vi "svx_Commit Hardware Settings (DAQmx).vi"(0 "acquisition task in":T1={"AI device settings"={"AI DAQmx TaskID"="", "response"=[]}, "acquisition type"=enum."Finite", "measurement settings"={"AI sampling frequency"=51200.0, "AO sampling frequency"=51200.0, "AI block size"=0, "AO block Size"=0, "block duration [ms]"=100.0, "number of AI channels"=0, "device propagation delay [samples]"=0.0, "DUT propagation time [s]"=0.0}, "settling settings"={"settle time"=0.015599999576807022, "settle cycles"=5}, "integration settings"={"integration time"=0.015599999576807022, "integration cycles"=5}, "AO device settings"={"AO DAQmx taskID"="", "excitation"=[]}, "acquisition accounting"={"initial read size [samples]"=0, "read offset [samples]"=0, "read length [samples]"=0, "blocks to settle [samples]"=0, "min delay until transition [samples]"=0}, "frequency range"={"start frequency"=0.015599999576807022, "stop frequency"=5.0}, "block type"=enum."Initialize", "source settings"={"signal type"=enum."Dual tone (IMD)", "frequency"=0.0, "total amplitude"=0.0, "frequencies"=[1.0], "relative amplitudes"=[1.0], "offset"=1.0, "total amplitude list"=[1.0], "ramping rate"=0.0}, "chirp settings"={"amplitude"=0.0, "frequency range"={"start (Hz)"=20.0, "stop (Hz)"=20000.0, "frequency spacing"=enum."Logarithmic"}, "sampling info"={"Fs"=50000.0, "chirp duration [s]"=3.0}, "initial states"={"frequency [Hz]"=20.0, "phase [rad]"=0.0, "elapsed time [s]"=0.0}, "frequency slope"=0.0, "maximum harmonic"=0, "prefix len [samples]"={"integer"=0, "fractional"=0.0}}} {"chirp settings"."frequency slope" format="%.2f"; "chirp settings"."prefix len [samples]"."fractional" format="%.2p"; "chirp settings"."initial states"."elapsed time [s]" format="%.2f"; "chirp settings"."initial states"."phase [rad]" format="%.2f"; "chirp settings"."initial states"."frequency [Hz]" format="%.2f"; "chirp settings"."sampling info"."chirp duration [s]" format="%.2f"; "chirp settings"."sampling info"."Fs" format="%.2p"; "chirp settings"."frequency range"."stop (Hz)" format="%.2f"; "chirp settings"."frequency range"."start (Hz)" format="%.2f"; "chirp settings"."amplitude" format="%.2f"; "source settings"."total amplitude" format="%.2f"; "source settings"."relative amplitudes" format="%.2f"; "source settings"."frequencies" format="%.2f"; "source settings"."total amplitude list" format="%.2f"; "source settings"."ramping rate" format="%.4f"; "source settings"."offset" format="%.2f"; "source settings"."frequency" format="%.2f"; "frequency range"."stop frequency" format="%.2f"; "frequency range"."start frequency" format="%.2f"; "AO device settings"."excitation"."AO channel settings"."terminal config" items=["Default"=-1, "Differential"=10106, "Pseudodifferential"=12529]; "AI device settings"."response"."AI channel settings"."DSA channel settings"."IEPE current [mA]" min=0.0 max=20.0 format="%.1f"; "AI device settings"."response"."AI channel settings"."DSA channel settings"."coupling" items=["AC"=10045, "DC"=10050, "GND"=10066]; "AI device settings"."response"."AI channel settings"."min value [V]" format="%.2f"; "AI device settings"."response"."AI channel settings"."terminal config" items=["Default"=-1, "RSE"=10083, "NRSE"=10078, "Differential"=10106, "Pseudodifferential"=12529]; "AI device settings"."response"."AI channel settings"."max value [V]" format="%.2f"; "integration settings"."integration time" format="%.2p"; "settling settings"."settle time" format="%.2p"; "measurement settings"."DUT propagation time [s]" format="%.2f"; "measurement settings"."AO sampling frequency" format="%.2f"; "measurement settings"."AI sampling frequency" format="%.2f"}, 11 "error in (no error)":errorcluster, 12 "block size limits":T5={"minimum block size"=50, "maximum block size"=131072}) -> (4 "acquisition task out":T1={"AI device settings"={"AI DAQmx TaskID"="", "response"=[{"AI physical channel"="Dev1/ai0", "AI channel settings"={"max value [V]"=10.0, "min value [V]"=10.0, "terminal config"=-1, "DSA channel settings"={"coupling"=10045, "enable IEPE excitation"=FALSE, "IEPE current [mA]"=4.0}}}]}, "acquisition type"=enum."Finite", "measurement settings"={"AI sampling frequency"=0.0, "AO sampling frequency"=0.0, "AI block size"=0, "AO block Size"=0, "block duration [ms]"=100.0, "number of AI channels"=0, "device propagation delay [samples]"=0.0, "DUT propagation time [s]"=0.0}, "settling settings"={"settle time"=0.015599999576807022, "settle cycles"=5}, "integration settings"={"integration time"=0.015599999576807022, "integration cycles"=5}, "AO device settings"={"AO DAQmx taskID"="", "excitation"=[{"AO physical channel"="Dev1/ao0", "AO channel settings"={"maximum value (10 V)"=10.0, "minimum value (10 V)"=-10.0, "terminal config"=-1}}]}, "acquisition accounting"={"initial read size [samples]"=0, "read offset [samples]"=0, "read length [samples]"=0, "blocks to settle [samples]"=0, "min delay until transition [samples]"=0}, "frequency range"={"start frequency"=-1.0, "stop frequency"=-1.0}, "block type"=enum."Initialize", "source settings"={"signal type"=enum."Sine wave", "frequency"=0.0, "total amplitude"=0.0, "frequencies"=[1.0], "relative amplitudes"=[1.0], "offset"=1.0, "total amplitude list"=[1.0], "ramping rate"=0.0}, "chirp settings"={"amplitude"=0.0, "frequency range"={"start (Hz)"=20.0, "stop (Hz)"=20000.0, "frequency spacing"=enum."Logarithmic"}, "sampling info"={"Fs"=50000.0, "chirp duration [s]"=3.0}, "initial states"={"frequency [Hz]"=20.0, "phase [rad]"=0.0, "elapsed time [s]"=0.0}, "frequency slope"=0.0, "maximum harmonic"=0, "prefix len [samples]"={"integer"=0, "fractional"=0.0}}} {"chirp settings"."frequency slope" format="%.2f"; "chirp settings"."prefix len [samples]"."fractional" format="%.2p"; "chirp settings"."initial states"."elapsed time [s]" format="%.2f"; "chirp settings"."initial states"."phase [rad]" format="%.2f"; "chirp settings"."initial states"."frequency [Hz]" format="%.2f"; "chirp settings"."sampling info"."chirp duration [s]" format="%.2f"; "chirp settings"."sampling info"."Fs" format="%.2p"; "chirp settings"."frequency range"."stop (Hz)" format="%.2f"; "chirp settings"."frequency range"."start (Hz)" format="%.2f"; "chirp settings"."amplitude" format="%.2f"; "source settings"."total amplitude" format="%.2f"; "source settings"."relative amplitudes" format="%.2f"; "source settings"."frequencies" format="%.2f"; "source settings"."total amplitude list" format="%.2f"; "source settings"."ramping rate" format="%.4f"; "source settings"."offset" format="%.2f"; "source settings"."frequency" format="%.2f"; "frequency range"."stop frequency" format="%.2f"; "frequency range"."start frequency" format="%.2f"; "AO device settings"."excitation"."AO channel settings"."terminal config" items=["Default"=-1, "Differential"=10106, "Pseudodifferential"=12529]; "AI device settings"."response"."AI channel settings"."DSA channel settings"."IEPE current [mA]" min=0.0 max=20.0 format="%.1f"; "AI device settings"."response"."AI channel settings"."DSA channel settings"."coupling" items=["AC"=10045, "DC"=10050, "GND"=10066]; "AI device settings"."response"."AI channel settings"."min value [V]" format="%.2f"; "AI device settings"."response"."AI channel settings"."terminal config" items=["Default"=-1, "RSE"=10083, "NRSE"=10078, "Differential"=10106, "Pseudodifferential"=12529]; "AI device settings"."response"."AI channel settings"."max value [V]" format="%.2f"; "integration settings"."integration time" format="%.2p"; "settling settings"."settle time" format="%.2p"; "measurement settings"."DUT propagation time [s]" format="%.2f"; "measurement settings"."AO sampling frequency" format="%.2f"; "measurement settings"."AI sampling frequency" format="%.2f"}, 13 "measurements per second":dbl format="%.2f", 14 "actual sample rate":dbl format="%.2f", 15 "error out":errorcluster)   [LabVIEW 2017]
doc: "This example VI commits the analog input and output tasks to perform an audio measurement on a DUT. Before calling <B>SVXMPL_Commit Hardware Settings (DAQmx).vi</B>, you should initialize and configure the measurment task using <B>SVXMPL_Initialize (DAQmx).vi</B>, <B>SVXMPL_Configure Source (DAQmx).vi</B>, <B>SVXMPL_Configure Measurement.vi</B>, and (if needed) <B>SVXMPL_Override DAQmx Parameters.vi</B>.\n\nThe only configuration input for this VI is the <B>block size limits</B> cluster. The block size, in samples, is dependent on input selections from <B>SVXMPL_Configure Measurement.vi</B> and <B>SVXMPL_Override DAQmx Parameters.vi</B>. If the block size defined in the task lies outside the <B>block size limits</B> it will be coerced into this range.\n\nThe VI returns the actual hardware sampling rate in samples per second as well as the time interval required for each integration period in the measurement."
uses:
  <vilib>/addons/Sound and Vibration/Example Support/Audio/DAQmx/svx_Acquisition Task (DAQmx).ctl
  <vilib>/addons/_NISVFA/_Shared subVIs/Controls/svc_Channel Settings.ctl
  <vilib>/addons/_NISVFA/_Shared subVIs/Controls/svc_DSA Channel Settings.ctl
  <vilib>/addons/_NISVFA/_Generation/subVIs/sv_Chirp Settings.ctl
  <vilib>/addons/_NISVFA/_Generation/SoundVib_Generation.lvlib
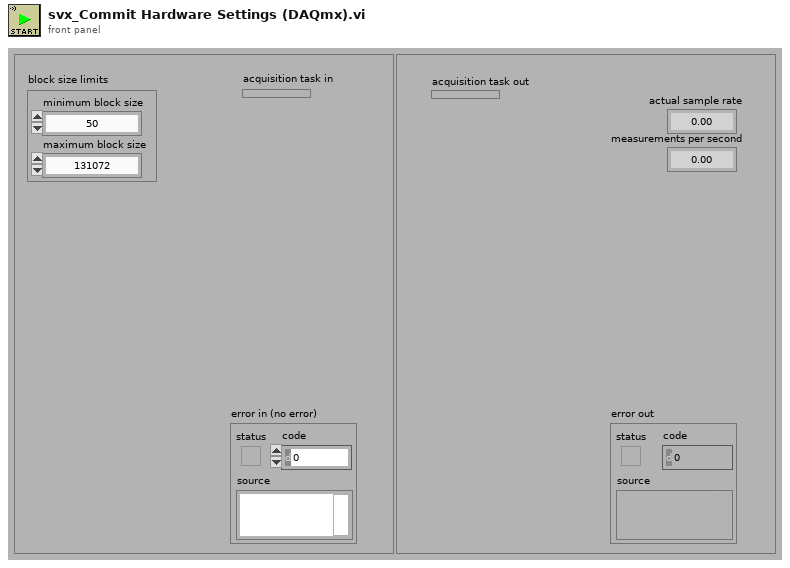
[diagram p1: front panel]
types:
  T1 = typedef "svx_Acquisition Task (DAQmx).ctl" = cluster{"AI device settings":cluster{"AI DAQmx TaskID":refnum<k21>, "response":cluster{"AI physical channel":tag, "AI channel settings":T2}[]}, "acquisition type":enum16{"Finite", "Averaged", "Settled", "Amplitude Sweep", "Stepped Frequency Sweep", "Continuous Frequency Sweep"}, "measurement settings":cluster{"AI sampling frequency":dbl, "AO sampling frequency":dbl, "AI block size":i32, "AO block Size":i32, "block duration [ms]":dbl, "number of AI channels":i32, "device propagation delay [samples]":dbl, "DUT propagation time [s]":dbl}, "settling settings":cluster{"settle time":dbl, "settle cycles":i32}, "integration settings":cluster{"integration time":dbl, "integration cycles":i32}, "AO device settings":cluster{"AO DAQmx taskID":refnum<k21>, "excitation":cluster{"AO physical channel":tag, "AO channel settings":cluster{"maximum value (10 V)":dbl, "minimum value (10 V)":dbl, "terminal config":i32}}[]}, "acquisition accounting":cluster{"initial read size [samples]":i32, "read offset [samples]":i32, "read length [samples]":i32, "blocks to settle [samples]":i32, "min delay until transition [samples]":i32}, "frequency range":cluster{"start frequency":dbl, "stop frequency":dbl}, "block type":enum16{"Initialize", "Settle", "Integrate"}, "source settings":cluster{"signal type":enum16{"Sine wave", "Dual tone (IMD)", "Multitone", "Chirp", "Frequency flat chirp", "Uniform white noise", "Gaussian white noise", "Pink noise", "PRN", "Continuous swept-sine"}, "frequency":dbl, "total amplitude":dbl, "frequencies":dbl[], "relative amplitudes":dbl[], "offset":dbl, "total amplitude list":dbl[], "ramping rate":dbl}, "chirp settings":T4}
  T2 = typedef "svc_Channel Settings.ctl" = cluster{"max value [V]":dbl, "min value [V]":dbl, "terminal config":i32, "DSA channel settings":T3}
  T3 = typedef "svc_DSA Channel Settings.ctl" = cluster{"coupling":i32, "enable IEPE excitation":bool, "IEPE current [mA]":dbl}
  T4 = typedef "SoundVib_Generation.lvlib/sv_Chirp Settings.ctl" = cluster{"amplitude":dbl, "frequency range":cluster{"start (Hz)":dbl, "stop (Hz)":dbl, "frequency spacing":enum16{"Linear", "Logarithmic"}}, "sampling info":cluster{"Fs":dbl, "chirp duration [s]":dbl}, "initial states":cluster{"frequency [Hz]":dbl, "phase [rad]":dbl, "elapsed time [s]":dbl}, "frequency slope":dbl, "maximum harmonic":i32, "prefix len [samples]":cluster{"integer":u32, "fractional":dbl}}
  T5 = cluster{"minimum block size":i32, "maximum block size":i32}
  T6 = enum16{"Finite", "Averaged", "Settled", "Amplitude Sweep", "Stepped Frequency Sweep", "Continuous Frequency Sweep"}
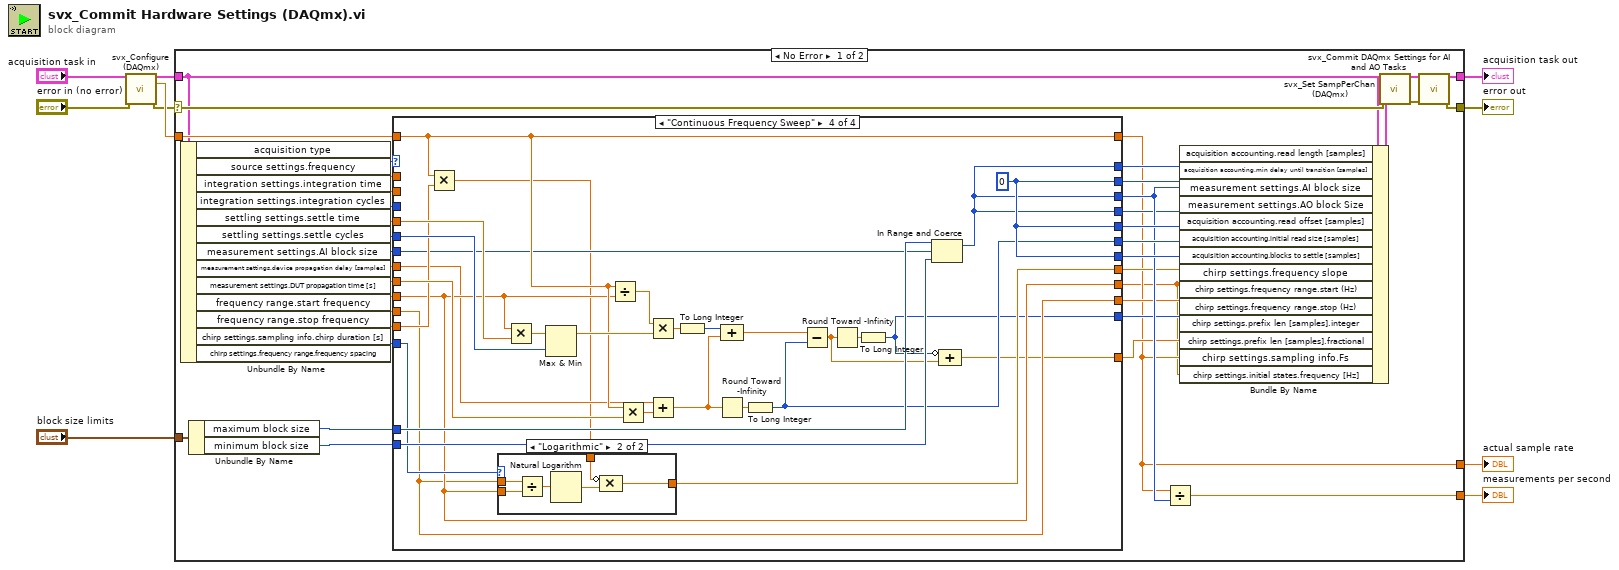
[diagram p0: block diagram]
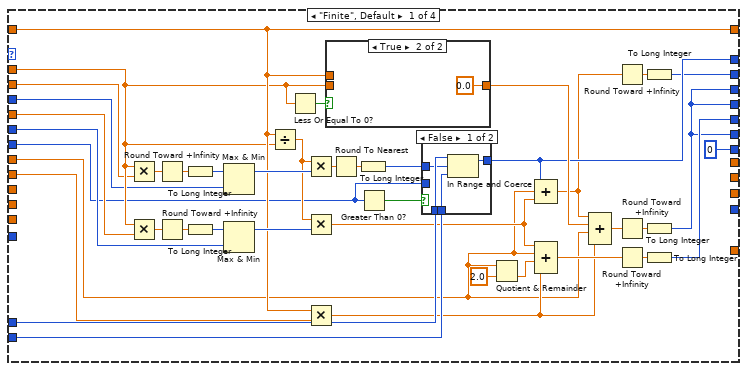
[diagram p2: hidden frame]
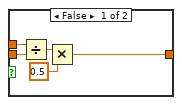
[diagram p4: hidden frame]
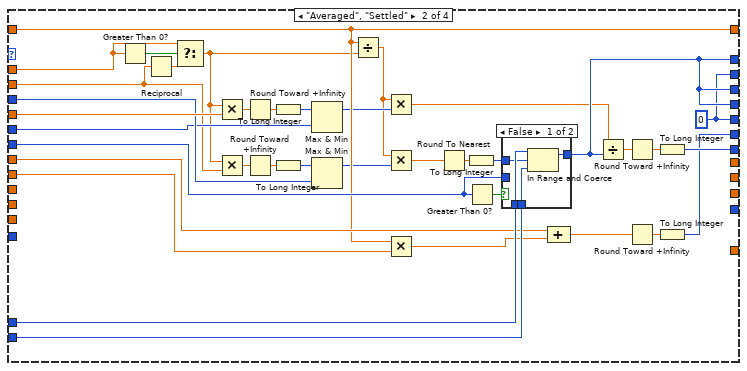
[diagram p5: hidden frame]
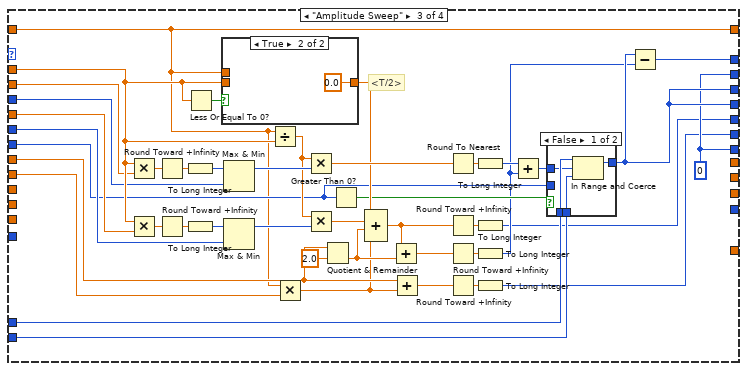
[diagram p7: hidden frame]
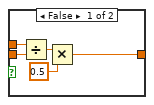
[diagram p9: hidden frame]
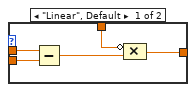
[diagram p10: hidden frame]
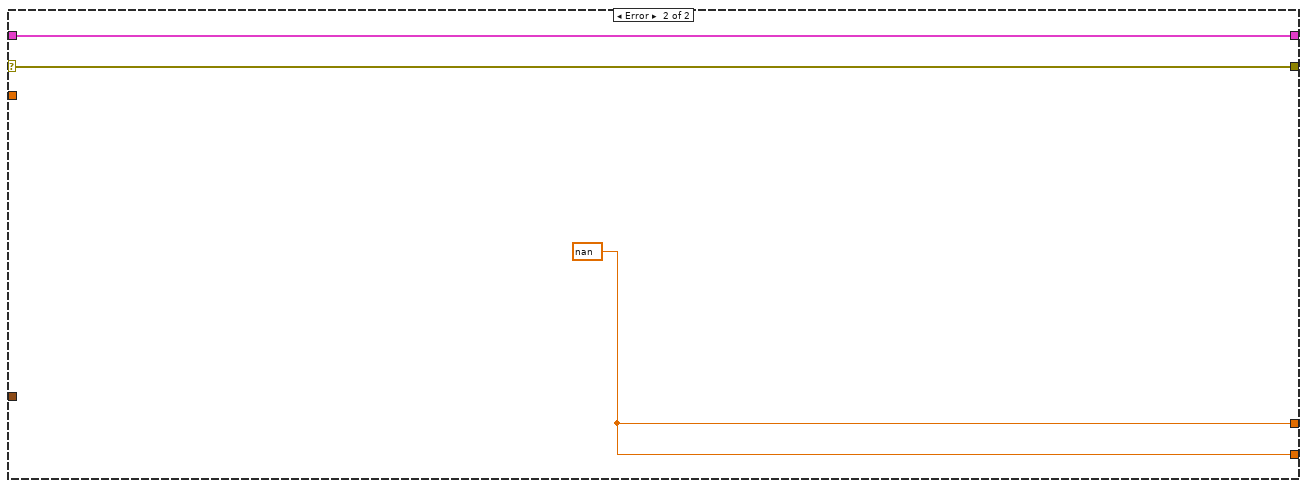
[diagram p11: hidden frame]
diagram:
  n1 = call <vilib>:"svx_Configure (DAQmx).vi"("acquisition task in"="acquisition task in", "error in (no error)"="error in (no error)") -> ("acquisition task out"=w4:T1, "actual scan rate"=w3:dbl, "error out"=w2:errorcluster)  [unwired: 11 in]
  n2 = case shown="No Error" w2 {
    selector: w2 -> [w27 w238]
    tunnel: w4 -> [w26 w240]
    tunnel: [w23 w240] -> w1
    tunnel: [w21 w238] -> w9
    tunnel: w3 -> [w30 _]
    tunnel: "block size limits" -> [w38 _]
    tunnel: [w31 w239] -> w6
    tunnel: [w12 w239] -> w5
    frame No Error {
      n3 = Unbundle By Name(w26) -> ("acquisition type"=w32:T6, "source settings.frequency"=w48:dbl, "integration settings.integration time"=w47:dbl, "integration settings.integration cycles"=w46:i32, "settling settings.settle time"=w45:dbl, "settling settings.settle cycles"=w44:i32, "measurement settings.AI block size"=w43:i32, "measurement settings.device propagation delay [samples]"=w42:dbl, "measurement settings.DUT propagation time [s]"=w41:dbl, "frequency range.start frequency"=w20:dbl, "frequency range.stop frequency"=w19:dbl, "chirp settings.sampling info.chirp duration [s]"=w18:dbl, "chirp settings.frequency range.frequency spacing"=w17:enum16{"Linear", "Logarithmic"})
      n4 = Unbundle By Name(w38) -> ("maximum block size"=w40:i32, "minimum block size"=w39:i32)
      n5 = case shown="\"Continuous Frequency Sweep\"" w32 {
        tunnel: w30 -> [w72 w113 w156 w217]
        tunnel: w48 -> [w68 w107 w167 _]
        tunnel: w47 -> [w67 w101 w166 _]
        tunnel: w46 -> [w66 w115 w165 _]
        tunnel: w45 -> [w65 w116 w164 w224]
        tunnel: w44 -> [w64 w114 w163 w223]
        tunnel: w43 -> [w63 w127 w162 w199]
        tunnel: w42 -> [w49 w132 w161 w209]
        tunnel: w41 -> [w62 w131 w160 w222]
        tunnel: w40 -> [w70 w134 w159 w221]
        tunnel: w39 -> [w69 w133 w158 w220]
        tunnel: [w72 w113 w156 w217] -> w12
        tunnel: [w71 w125 w157 w211] -> w37
        tunnel: [w56 w123 w154 w212] -> w36
        tunnel: [w53 w125 w155 w211] -> w29
        tunnel: [w53 w125 w155 w211] -> w28
        tunnel: [w58 w123 w145 w212] -> w35
        tunnel: [w53 w103 w151 w207] -> w34
        tunnel: [0 ("acquisition accounting.min delay until transition [samples]") w128 w154 w212] -> w33
        tunnel: w20 -> [_ _ _ w213]
        tunnel: w19 -> [_ _ _ w210]
        tunnel: w18 -> [_ _ _ w216]
        tunnel: w17 -> [_ _ _ w215]
        tunnel: [_ _ _ w214] -> w16
        tunnel: [_ _ _ w213] -> w11
        tunnel: [_ _ _ w210] -> w15
        tunnel: [_ _ _ w204] -> w13
        tunnel: [_ _ _ w198] -> w14
        frame "Finite", Default {
          n6 = Multiply(x=w68, y=w67) -> (x*y=w80:dbl)
          n7 = Multiply(x=w68, y=w65) -> (x*y=w78:dbl)
          n8 = Round Toward +Infinity(x=w80) -> (ceil(x): smallest int >= x=w81:dbl)
          n9 = Round Toward +Infinity(x=w78) -> (ceil(x): smallest int >= x=w77:dbl)
          n10 = To Long Integer(number=w81) -> (32bit integer=w82:i32)
          n11 = To Long Integer(number=w77) -> (32bit integer=w76:i32)
          n12 = Max & Min(x=w82, y=w66) -> (max(x,y)=w79:i32)  [unwired: 1 out]
          n13 = Max & Min(x=w76, y=w64) -> (max(x,y)=w75:i32)  [unwired: 1 out]
          n14 = Divide(x=w72, y=w68) -> (x/y=w74:dbl)
          n15 = Less Or Equal To 0?(x=w68) -> (x <= 0?=w89:bool)
          n16 = Multiply(x=w74, y=w79) -> (x*y=w85:dbl)
          n17 = Multiply(x=w74, y=w75) -> (x*y=w52:dbl)
          n18 = Multiply(x=w72, y=w62) -> (x*y=w51:dbl)
          n19 = case shown="True" w89 {
            tunnel: [w95 0.0] -> w84
            tunnel: w72 -> [w98 _]
            tunnel: w68 -> [w96 _]
            frame False {
              n20 = Divide(x=w98, y=w96) -> (x/y=w99:dbl)
              n21 = Multiply(x=w99, y=0.5) -> (x*y=w95:dbl)
            }
            frame True {
            }
          }
          n22 = Round To Nearest(number=w85) -> (nearest integer value=w86:dbl)
          n23 = To Long Integer(number=w86) -> (32bit integer=w88:i32)
          n24 = Greater Than 0?(x=w63) -> (x > 0?=w87:bool)
          n25 = case shown="False" w87 {
            tunnel: w88 -> [w91 _]
            tunnel: w63 -> [_ w94]
            tunnel: [w90 w94] -> w71
            tunnel: w70 -> [w93 _]
            tunnel: w69 -> [w92 _]
            frame False {
              n26 = In Range and Coerce(upper limit=w93, x=w91, lower limit=w92) -> (coerced(x)=w90:i32)  [unwired: 1 out]
            }
            frame True {
            }
          }
          n27 = Quotient & Remainder(x=w49, y=2.0) -> (floor(x/y)=w73:dbl)  [unwired: 1 out]
          n28 = Compound Arithmetic op=ADD(w71, w49, w52) -> (w50:dbl)
          n29 = Compound Arithmetic op=ADD(w52, w49, w73, w51) -> (w59:dbl)
          n30 = Compound Arithmetic op=ADD(w50, w84, w49, w51) -> (w54:dbl)
          n31 = Round Toward +Infinity(x=w50) -> (ceil(x): smallest int >= x=w57:dbl)
          n32 = Round Toward +Infinity(x=w54) -> (ceil(x): smallest int >= x=w55:dbl)
          n33 = Round Toward +Infinity(x=w59) -> (ceil(x): smallest int >= x=w60:dbl)
          n34 = To Long Integer(number=w57) -> (32bit integer=w56:i32)
          n35 = To Long Integer(number=w55) -> (32bit integer=w53:i32)
          n36 = To Long Integer(number=w60) -> (32bit integer=w58:i32)
        }
        frame "Averaged", "Settled" {
          w123 = 0
          n37 = Greater Than 0?(x=w107) -> (x > 0?=w109:bool)
          n38 = Reciprocal(x=w101) -> (1/x=w106:dbl)
          n39 = Select(t=w107, s=w109, f=w106) -> (s? t:f=w108:dbl)
          n40 = Multiply(x=w108, y=w116) -> (x*y=w119:dbl)
          n41 = Multiply(x=w108, y=w101) -> (x*y=w120:dbl)
          n42 = Round Toward +Infinity(x=w119) -> (ceil(x): smallest int >= x=w118:dbl)
          n43 = Round Toward +Infinity(x=w120) -> (ceil(x): smallest int >= x=w121:dbl)
          n44 = To Long Integer(number=w118) -> (32bit integer=w117:i32)
          n45 = To Long Integer(number=w121) -> (32bit integer=w122:i32)
          n46 = Max & Min(x=w117, y=w114) -> (max(x,y)=w112:i32)  [unwired: 1 out]
          n47 = Max & Min(x=w122, y=w115) -> (max(x,y)=w111:i32)  [unwired: 1 out]
          n48 = Divide(x=w113, y=w108) -> (x/y=w110:dbl)
          n49 = Multiply(x=w110, y=w112) -> (x*y=w124:dbl)
          n50 = Multiply(x=w110, y=w111) -> (x*y=w126:dbl)
          n51 = Multiply(x=w113, y=w131) -> (x*y=w102:dbl)
          n52 = Round To Nearest(number=w126) -> (nearest integer value=w135:dbl)
          n53 = To Long Integer(number=w135) -> (32bit integer=w137:i32)
          n54 = Greater Than 0?(x=w127) -> (x > 0?=w136:bool)
          n55 = case shown="False" w136 {
            tunnel: w137 -> [w139 _]
            tunnel: w127 -> [_ w142]
            tunnel: [w138 w142] -> w125
            tunnel: w134 -> [w141 _]
            tunnel: w133 -> [w140 _]
            frame False {
              n56 = In Range and Coerce(upper limit=w141, x=w139, lower limit=w140) -> (coerced(x)=w138:i32)  [unwired: 1 out]
            }
            frame True {
            }
          }
          n57 = Compound Arithmetic op=ADD(w132, w102) -> (w104:dbl)
          n58 = Divide(x=w124, y=w125) -> (x/y=w129:dbl)
          n59 = Round Toward +Infinity(x=w129) -> (ceil(x): smallest int >= x=w130:dbl)
          n60 = Round Toward +Infinity(x=w104) -> (ceil(x): smallest int >= x=w105:dbl)
          n61 = To Long Integer(number=w130) -> (32bit integer=w128:i32)
          n62 = To Long Integer(number=w105) -> (32bit integer=w103:i32)
        }
        frame "Amplitude Sweep" {
          w154 = 0 ("acquisition accounting.min delay until transition [samples]")
          # "<T/2>"
          n63 = Multiply(x=w167, y=w166) -> (x*y=w179:dbl)
          n64 = Multiply(x=w167, y=w164) -> (x*y=w177:dbl)
          n65 = Round Toward +Infinity(x=w179) -> (ceil(x): smallest int >= x=w180:dbl)
          n66 = Round Toward +Infinity(x=w177) -> (ceil(x): smallest int >= x=w176:dbl)
          n67 = To Long Integer(number=w180) -> (32bit integer=w181:i32)
          n68 = To Long Integer(number=w176) -> (32bit integer=w175:i32)
          n69 = Less Or Equal To 0?(x=w167) -> (x <= 0?=w185:bool)
          n70 = case shown="True" w185 {
            tunnel: [w191 0.0] -> w171
            tunnel: w156 -> [w194 _]
            tunnel: w167 -> [w192 _]
            frame False {
              n71 = Divide(x=w194, y=w192) -> (x/y=w195:dbl)
              n72 = Multiply(x=w195, y=0.5) -> (x*y=w191:dbl)
            }
            frame True {
            }
          }
          n73 = Max & Min(x=w181, y=w165) -> (max(x,y)=w178:i32)  [unwired: 1 out]
          n74 = Max & Min(x=w175, y=w163) -> (max(x,y)=w174:i32)  [unwired: 1 out]
          n75 = Divide(x=w156, y=w167) -> (x/y=w173:dbl)
          n76 = Multiply(x=w156, y=w160) -> (x*y=w143:dbl)
          n77 = Multiply(x=w173, y=w178) -> (x*y=w183:dbl)
          n78 = Multiply(x=w173, y=w174) -> (x*y=w144:dbl)
          n79 = Quotient & Remainder(x=w161, y=2.0) -> (floor(x/y)=w168:dbl)  [unwired: 1 out]
          n80 = Greater Than 0?(x=w162) -> (x > 0?=w169:bool)
          n81 = Compound Arithmetic op=ADD(w171, w144, w168, w143) -> (w146:dbl)
          n82 = Add(x=w146, y=w168) -> (x+y=w149:dbl)
          n83 = Add(x=w161, y=w143) -> (x+y=w152:dbl)
          n84 = Round To Nearest(number=w183) -> (nearest integer value=w184:dbl)
          n85 = Round Toward +Infinity(x=w146) -> (ceil(x): smallest int >= x=w147:dbl)
          n86 = Round Toward +Infinity(x=w149) -> (ceil(x): smallest int >= x=w150:dbl)
          n87 = Round Toward +Infinity(x=w152) -> (ceil(x): smallest int >= x=w153:dbl)
          n88 = To Long Integer(number=w184) -> (32bit integer=w172:i32)
          n89 = To Long Integer(number=w147) -> (32bit integer=w145:i32)
          n90 = To Long Integer(number=w150) -> (32bit integer=w148:i32)
          n91 = To Long Integer(number=w153) -> (32bit integer=w151:i32)
          n92 = Add(x=w172, y=w148) -> (x+y=w170:i32)
          n93 = case shown="False" w169 {
            tunnel: w170 -> [w187 _]
            tunnel: w162 -> [_ w190]
            tunnel: [w186 w190] -> w155
            tunnel: w159 -> [w189 _]
            tunnel: w158 -> [w188 _]
            frame False {
              n94 = In Range and Coerce(upper limit=w189, x=w187, lower limit=w188) -> (coerced(x)=w186:i32)  [unwired: 1 out]
            }
            frame True {
            }
          }
          n95 = Subtract(x=w155, y=w148) -> (x-y=w157:i32)
        }
        frame "Continuous Frequency Sweep" {
          w212 = 0 ("acquisition accounting.min delay until transition [samples]")
          n96 = Multiply(x=w217, y=w216) -> (x*y=w197:dbl)
          n97 = case shown="\"Logarithmic\"" w215 {
            tunnel: w210 -> [w230 w237]
            tunnel: w197 -> [w228 w234]
            tunnel: w213 -> [w231 w233]
            tunnel: [w227 w232] -> w214
            frame "Linear", Default {
              n98 = Subtract(x=w230, y=w231) -> (x-y=w229:dbl)
              n99 = Compound Arithmetic op=MULTIPLY(invert w228, w229) -> (w227:dbl)
            }
            frame "Logarithmic" {
              n100 = Divide(x=w237, y=w233) -> (x/y=w236:dbl)
              n101 = Natural Logarithm(1:w236) -> (0:w235:dbl)
              n102 = Compound Arithmetic op=MULTIPLY(invert w234, w235) -> (w232:dbl)
            }
          }
          n103 = Multiply(x=w213, y=w224) -> (x*y=w201:dbl)
          n104 = Max & Min(x=w201, y=w223) -> (max(x,y)=w226:dbl)  [unwired: 1 out]
          n105 = Divide(x=w217, y=w213) -> (x/y=w225:dbl)
          n106 = Multiply(x=w217, y=w222) -> (x*y=w218:dbl)
          n107 = Multiply(x=w225, y=w226) -> (x*y=w206:dbl)
          n108 = Add(x=w209, y=w218) -> (x+y=w208:dbl)
          n109 = To Long Integer(number=w206) -> (32bit integer=w200:i32)
          n110 = Round Toward -Infinity(1:w208) -> (0:w219:dbl)
          n111 = Compound Arithmetic op=ADD(w200, w208) -> (w203:dbl)
          n112 = To Long Integer(number=w219) -> (32bit integer=w207:i32)
          n113 = Subtract(x=w203, y=w207) -> (x-y=w205:dbl)
          n114 = Round Toward -Infinity(1:w205) -> (0:w202:dbl)
          n115 = To Long Integer(number=w202) -> (32bit integer=w198:i32)
          n116 = In Range and Coerce(upper limit=w221, x=w199, lower limit=w220) -> (coerced(x)=w211:i32)  [unwired: 1 out]
          n117 = Compound Arithmetic op=ADD(invert w198, w205) -> (w204:dbl)
        }
      }
      n118 = Divide(x=w12, y=w29) -> (x/y=w31:dbl)
      n119 = Bundle By Name(cluster=w26, "acquisition accounting.read length [samples]"=w37, "acquisition accounting.min delay until transition [samples]"=w36, "measurement settings.AI block size"=w29, "measurement settings.AO block Size"=w28, "acquisition accounting.read offset [samples]"=w35, "acquisition accounting.initial read size [samples]"=w34, "acquisition accounting.blocks to settle [samples]"=w33, "chirp settings.frequency slope"=w16, "chirp settings.frequency range.start (Hz)"=w11, "chirp settings.frequency range.stop (Hz)"=w15, "chirp settings.prefix len [samples].integer"=w14, "chirp settings.prefix len [samples].fractional"=w13, "chirp settings.sampling info.Fs"=w12, "chirp settings.initial states.frequency [Hz]"=w11) -> (w25:T1)
      n120 = call <vilib>:"svx_Set SampPerChan (DAQmx).vi"("acquisition task in"=w25, "error in (no error)"=w27) -> ("acquisition task out"=w24:T1, "error out"=w22:errorcluster)  [unwired: 12 in]
      n121 = call <vilib>:"svx_Commit DAQmx Settings for AI and AO Tasks.vi"("acquisition task in"=w24, "error in (no error)"=w22) -> ("acquisition task out"=w23:T1, "error out"=w21:errorcluster)  [unwired: 12 in]
    }
    frame Error {
      w239 = nan
    }
  }
  "error out" <- w9
  "measurements per second" <- w6
  "actual sample rate" <- w5
  "acquisition task out" <- w1
